vi "parse tcp plotter.vi"(9 "data in":string, 10 "shot #":string) -> (2 "variable values":string[](array[string]), 3 "shot # out":string)   [LabVIEW 2013]
panel:
  out "Variable names (inc device)":string[](array[string])
  out "Device Name":string
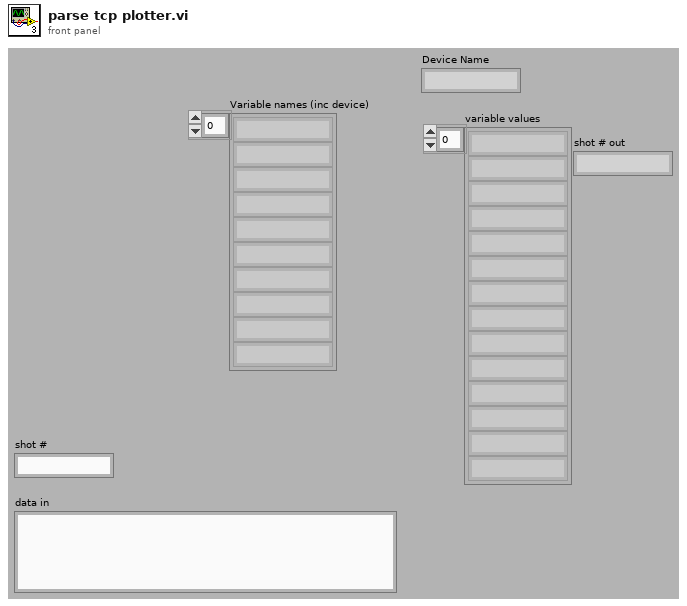
[diagram p1: front panel]
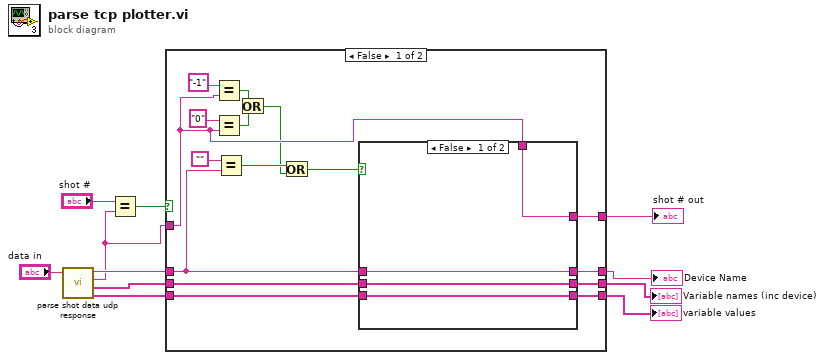
[diagram p0: block diagram]
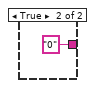
[diagram p2: hidden frame]
diagram:
  n1 = call "parse shot data udp response.vi"("ShotData UDP response"="data in") -> ("variable values"=w10:string[], "Variable names (inc device)"=w9:string[], "shot #"=w6:string, "Device Name"=w11:string)  [unwired: 2 in, 2 out]
  n2 = Equal?(x="shot #", y=w6) -> (x = y?=w5:bool)
  n3 = case shown="False" w5 {
    tunnel: w11 -> [w24 _]
    tunnel: w10 -> [w22 _]
    tunnel: w9 -> [w21 _]
    tunnel: w6 -> [w15 _]
    tunnel: [w20 _] -> w4
    tunnel: [w19 _] -> w3
    tunnel: [w18 _] -> w2
    tunnel: [w17 _] -> w1
    frame False {
      n4 = Equal?(x="-1", y=w15) -> (x = y?=w14:bool)
      n5 = Equal?(x="0", y=w15) -> (x = y?=w13:bool)
      n6 = Equal?(x="", y=w24) -> (x = y?=w26:bool)
      n7 = Or(x=w14, y=w13) -> (x .or. y?=w12:bool)
      n8 = Or(x=w26, y=w12) -> (x .or. y?=w27:bool)
      n9 = case shown="False" w27 {
        tunnel: w24 -> [w31 _]
        tunnel: w21 -> [w29 _]
        tunnel: w22 -> [w30 _]
        tunnel: [w31 _] -> w20
        tunnel: [w30 _] -> w19
        tunnel: [w29 _] -> w18
        tunnel: [w28 "0" ("x")] -> w17
        tunnel: w15 -> [w28 _]
        frame False {
        }
        frame True {
        }
      }
    }
    frame True {
    }
  }
  "Device Name" <- w4
  "Variable names (inc device)" <- w2
  "variable values" <- w3
  "shot # out" <- w1
